vi "FUG_PowerSupply.Read_DB.vi"(0 "i ref in":refnum<vi>, 5 "error in (no error)":errorcluster) -> (14 "i ref out":refnum<vi>, 19 "error out (no error)":errorcluster)   [LabVIEW 2014, in "FUG_PowerSupply.lvlib"]
doc: "This VI reads outall important Values from the Database (or directly from the Baseprocess Class)"
uses:
  FUG_PowerSupply.lvlib
  CS_Core/BaseProcess/BaseProcess.lvlib
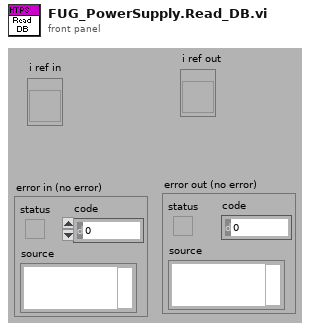
[diagram p1: front panel]
types:
  T1 = typedef "BaseProcess.lvlib/BaseProcess.i attribute.ctl" = cluster{"EventStatus":string, "EventError":i32, "PresetEvtWatchD":i32, "PresetPdcWatchD":i32, "EventTimeout":i32, "PeriodicInterval":i32, "Interface":string[], "Address":string[], "Special":string[], "PeriodicError":i32, "PeriodicStatus":string, "SuperProc":string, "Descriptors":T2[], "CaseRef":refnum<vi>, "PdcRef":refnum<vi>, "Thread Ref":refnum<vi>, "eventErrorID":i32, "eventStatusID":i32, "periodicErrorID":i32, "periodicStatusID":i32, "pdcCtrID":i32}
  T2 = typedef "BaseProcess.lvlib/BaseProcess.descriptor definition.ctl" = cluster{"selector":string, "descriptor":T3}
  T3 = typedef "BaseProcess.lvlib/BaseProcess.descriptor string definition.ctl" = string
  T4 = typedef "FUG_PowerSupply.lvlib/FUG_PowerSupply.i attribute.ctl" = cluster{"Type":string, "Elektrode Name":string, "CALC_FACTOR_SET_VOLTAGE":dbl, "CALC_FACTOR_GET_VOLTAGE":dbl, "CALC_FACTOR_GET_CURRENT":dbl, "CALC_FACTOR_SET_CURRENT ":dbl, "REG_VALUE":dbl, "Sign":bool, "setVoltID":i32, "setCurrentID":i32, "setPowerOnID":i32, "MaxVoltage":dbl}
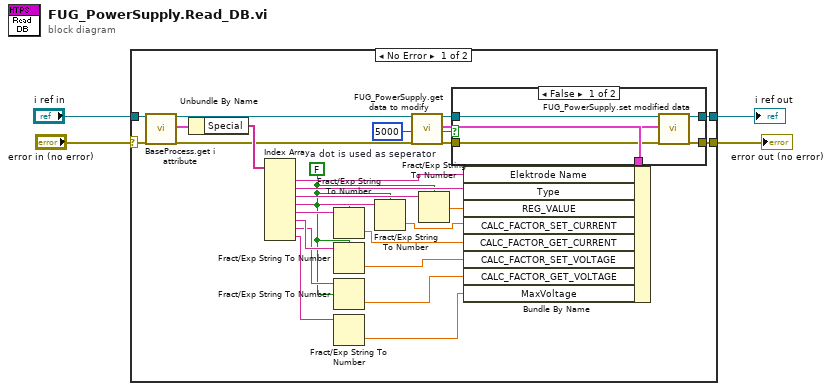
[diagram p0: block diagram]
diagram:
  n1 = case shown="No Error" "error in (no error)" {
    selector: "error in (no error)" -> [w29 w42]
    tunnel: [w32 w42] -> w1
    tunnel: "i ref in" -> [w31 w41]
    tunnel: [w33 w41] -> w3
    frame No Error {
      w9 = FALSE  # a dot is used as seperator
      n2 = call "BaseProcess.get i attribute.vi"("i ref in"=w31, "error in (no error)"=w29) -> ("i ref out"=w30:refnum<vi>, "i attribute"=w22:T1, "error out"=w18:errorcluster)  [unwired: 15 in]
      n3 = Unbundle By Name(w22) -> ("Special"=w21:string[])
      n4 = Index Array(array=w21) -> (element #1=w17:string, element #2=w16:string, element #3=w15:string, element #4=w14:string, element #5=w13:string, element #6=w12:string, element #7=w10:string, element #8=w5:string)  [unwired: 8 in]
      n5 = Fract/Exp String To Number(use system decimal point (T)=w9, string=w13) -> (number=w24:dbl)  [unwired: 2 in, 1 out]
      n6 = Fract/Exp String To Number(use system decimal point (T)=w9, string=w12) -> (number=w11:dbl)  [unwired: 2 in, 1 out]
      n7 = Fract/Exp String To Number(use system decimal point (T)=w9, string=w10) -> (number=w23:dbl)  [unwired: 2 in, 1 out]
      n8 = Fract/Exp String To Number(string=w5) -> (number=w6:dbl)  [unwired: 3 in, 1 out]
      n9 = Fract/Exp String To Number(use system decimal point (T)=w9, string=w14) -> (number=w25:dbl)  [unwired: 2 in, 1 out]
      n10 = call "FUG_PowerSupply.get data to modify.vi"("i ref in"=w30, "ms timeout (10000)"=5000, "error in (no error)"=w18) -> ("i ref out"=w28:refnum<vi>, "i attribute"=w20:T4, "timed out"=w8:bool, "error out"=w27:errorcluster)  [unwired: 13 in]
      n11 = Fract/Exp String To Number(use system decimal point (T)=w9, string=w15) -> (number=w26:dbl)  [unwired: 2 in, 1 out]
      n12 = Bundle By Name(cluster=w20, "Elektrode Name"=w17, "Type"=w16, "REG_VALUE"=w26, "CALC_FACTOR_SET_CURRENT"=w25, "CALC_FACTOR_GET_CURRENT"=w24, "CALC_FACTOR_SET_VOLTAGE"=w11, "CALC_FACTOR_GET_VOLTAGE"=w23, "MaxVoltage"=w6) -> (w19:T4)
      n13 = case shown="False" w8 {
        tunnel: [w38 w40] -> w33
        tunnel: [w37 w39] -> w32
        tunnel: w28 -> [w36 w40]
        tunnel: w27 -> [w35 w39]
        tunnel: w19 -> [w34 _]
        frame False {
          n14 = call "FUG_PowerSupply.set modified data.vi"("i ref in"=w36, "i attribute"=w34, "error in (no error)"=w35) -> ("i ref out"=w38:refnum<vi>, "error out"=w37:errorcluster)  [unwired: 15 in]
        }
        frame True {
        }
      }
    }
    frame Error {
    }
  }
  "error out (no error)" <- w1
  "i ref out" <- w3
